vi "pre-allocated_no_IPE.vi"(8 "error in (no error)":errorcluster, 11 "Test Data in":T1) -> (0 "error out":errorcluster, 3 "Test Data out":T1)   [LabVIEW 2024, in "Tester.lvlib"]
uses:
  Tester.lvlib
  test_data--cluster.ctl
  packetized_data--cluster.ctl
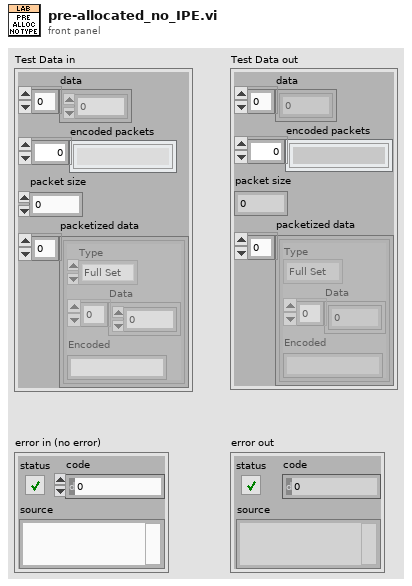
[diagram p1: front panel]
types:
  T1 = typedef "Tester.lvlib/test_data--cluster.ctl" = cluster{"data":dbl[], "encoded packets":string[], "packet size":i32, "packetized data":T2[]}
  T2 = typedef "Tester.lvlib/packetized_data--cluster.ctl" = cluster{"Type":enum16{"Full Set", "Last Set"}, "Data":dbl[], "Encoded":string}
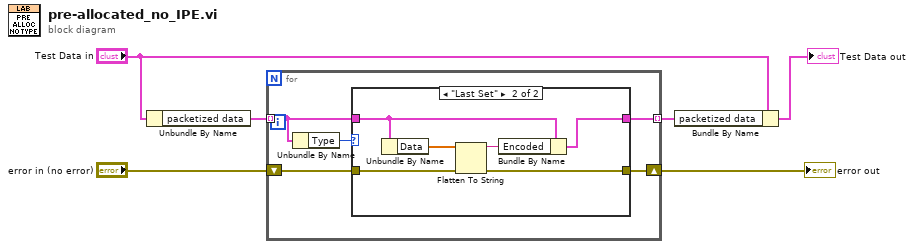
[diagram p0: block diagram]
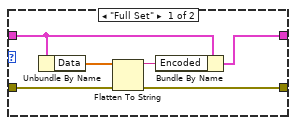
[diagram p2: hidden frame]
diagram:
  n1 = Unbundle By Name("Test Data in") -> ("packetized data"=w2:T2[])
  n2 = for {
    shift-right: [w11] -> w3
    shift-left: "error in (no error)" -> [w10]
    tunnel: w2 -> [w8] mode=indexing
    tunnel: [w7] -> w1 mode=indexing
    n3 = Unbundle By Name(w8) -> ("Type"=w9:enum16{"Full Set", "Last Set"})
    n4 = case shown="\"Last Set\"" w9 {
      tunnel: w8 -> [w17 w23]
      tunnel: [w16 w22] -> w11
      tunnel: w10 -> [w15 w21]
      tunnel: [w14 w20] -> w7
      frame "Full Set" {
        n5 = Unbundle By Name(w17) -> ("Data"=w13:dbl[])
        n6 = Flatten To String(anything=w13, error in (no error)=w15) -> (data string=w12:string, error out=w16:errorcluster)  [unwired: 2 in, 1 out]
        n7 = Bundle By Name(cluster=w17, "Encoded"=w12) -> (w14:T2)
      }
      frame "Last Set" {
        n8 = Unbundle By Name(w23) -> ("Data"=w19:dbl[])
        n9 = Flatten To String(anything=w19, error in (no error)=w21) -> (data string=w18:string, error out=w22:errorcluster)  [unwired: 2 in, 1 out]
        n10 = Bundle By Name(cluster=w23, "Encoded"=w18) -> (w20:T2)
      }
    }
  }
  "error out" <- w3
  n11 = Bundle By Name(cluster="Test Data in", "packetized data"=w1) -> (→"Test Data out":T1)
